vi "VIP Check.vi"(6 "Dev Mode":bool, 7 "Force Check(F)":bool, 8 "error in":errorcluster, 10 "Home version":bool, 11 "Product Name":string) -> (0 "error out":errorcluster, 1 "available version":string, 2 "Update available":bool, 3 "Continue":bool, 4 "Check Version":bool, 5 "current version":string)   [LabVIEW 2014, in "Raspberry Pi Compatible Compiler for LabVIEW.lvlib"]
uses:
  Raspberry Pi Compatible Compiler for LabVIEW.lvlib
  RasPi_Services/Download/RasPiDownloader.lvlib
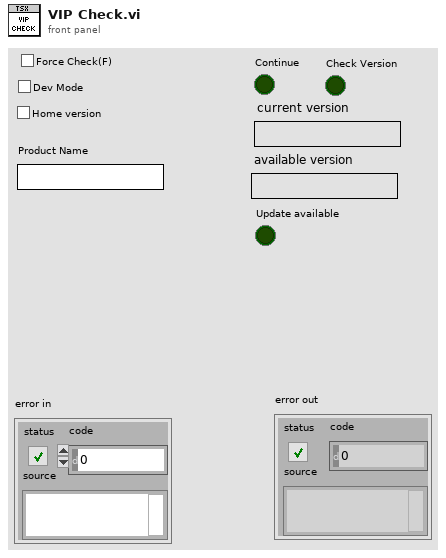
[diagram p1: front panel]
types:
  T1 = typedef "Raspberry Pi Compatible Compiler for LabVIEW.lvlib/RasPiDownloader.lvlib/RuntimeVersion.ctl" = cluster{"Major":i32, "Minor":i32, "Build":i32, "Revision":i32}
  T2 = typedef "Raspberry Pi Compatible Compiler for LabVIEW.lvlib/GitHub API.lvlib/GitHubContents_TD.ctl" = cluster{"name":string, "path":string, "sha":string, "size":dbl, "url":string, "html_url":string, "git_url":string, "download_url":string, "type":string, "_links":cluster{"self":string, "git":string, "html":string}}
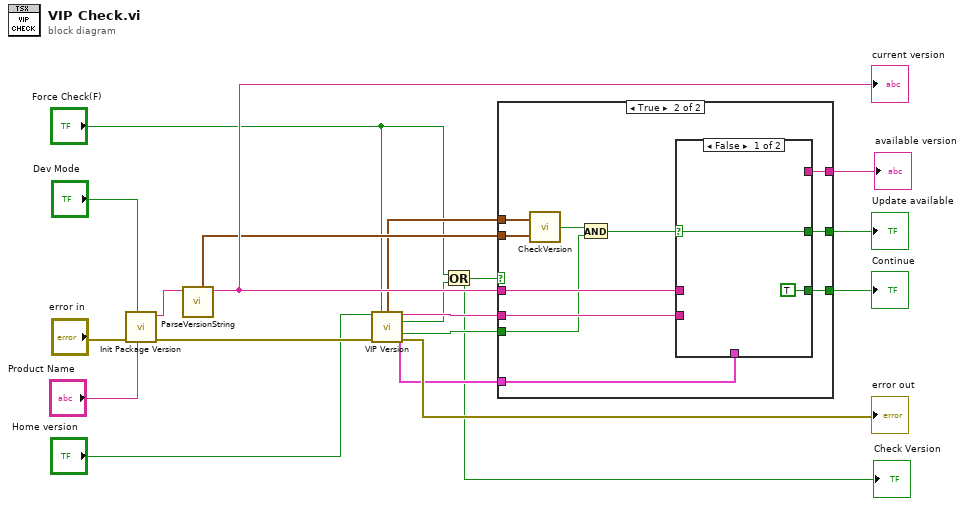
[diagram p0: block diagram]
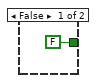
[diagram p2: hidden frame]
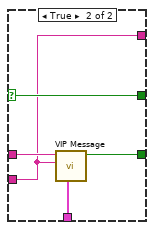
[diagram p3: hidden frame]
diagram:
  n1 = call "Init Package Version.vi"("Product Name"="Product Name", "Dev Mode"="Dev Mode", "error in"="error in") -> ("error out"=w16:errorcluster, "VIP Package Version"=w13:string)  [unwired: 7 in]
  n2 = call "ParseVersionString.vi"("version string"=w13) -> ("fixed version string"=w12:string, "Version"=w11:T1)  [unwired: 7 in]
  "current version" <- w12
  n3 = call "VIP Version.vi"("Home version"="Home version", "Force Check(F)"="Force Check(F)", "error in"=w16) -> ("Version"=w5:T1, "VIP version"=w7:string, "Check Version"=w2:bool, "Latest"=w6:T2, "Found"=w4:bool, "error out"=→"error out":errorcluster)  [unwired: 7 in]
  n4 = Or(x="Force Check(F)", y=w2) -> (x .or. y?=w3:bool)
  "Check Version" <- w3
  n5 = case shown="True" w3 {
    tunnel: [FALSE ("Continue") w31] -> w19
    tunnel: w12 -> [_ w30]
    tunnel: w11 -> [_ w29]
    tunnel: [_ w28] -> w9
    tunnel: [_ w27] -> w8
    tunnel: w7 -> [_ w26]
    tunnel: w6 -> [_ w25]
    tunnel: w5 -> [_ w24]
    tunnel: w4 -> [_ w22]
    frame False {
    }
    frame True {
      n6 = call "CheckVersion.vi"("Current Version"=w29, "New Version"=w24) -> ("update"=w23:bool)
      n7 = And(x=w23, y=w22) -> (x .and. y?=w21:bool)
      n8 = case shown="False" w21 {
        selector: w21 -> [w32 w35]
        tunnel: [TRUE ("Continue") w38] -> w31
        tunnel: w26 -> [_ w34]
        tunnel: w25 -> [_ w37]
        tunnel: w30 -> [_ w36]
        tunnel: [w32 w35] -> w28
        tunnel: [_ w34] -> w27
        frame False {
        }
        frame True {
          n9 = call "VIP Message.vi"("Latest VIP"=w37, "Latest Version"=w34, "Current Version"=w36) -> ("Continue"=w38:bool)  [unwired: 6 in]
        }
      }
    }
  }
  "Continue" <- w19
  "Update available" <- w9
  "available version" <- w8
